vi "boom_monitoring.vi"() -> ()   [LabVIEW 2020]
uses:
  <vilib>/DAQmx/read.llb/DAQmx Read (Analog 1D DBL NChan 1Samp).vi
  <vilib>/DAQmx/create/channels.llb/DAQmx Create Channel (AI-Voltage-Basic).vi
  sub_vi/Timing.llb/getRelativeTime(Host).vi
  <vilib>/DAQmx/miscellaneous.llb/DAQmx Fill In Error Info.vi
  sub_vi/Timing.llb/Timing.lvlib
panel:
  out "error out":errorcluster
  out "logging_state":bool
  in  "logging_cmd":bool
  in  "state":bool
  out "angle_Array":dbl[](array[numeric])
  out "getRelativeTime(sec)":dbl
  out "Waveform Chart":T1(graph)
  in  "zero_set":bool
  in  "Cluster":T2
  out "force":dbl format="%.2f"
  out "displacement":dbl format="%.1f"
  in  "stop":bool
  out "Boolean 6":bool
  out "Boolean 5":bool
  out "Boolean 4":bool
  out "Boolean 3":bool
  out "Boolean 2":bool
  out "Boolean":bool
  out "Angle_7":dbl format="%.1f"
  out "Angle_6":dbl format="%.1f"
  out "Angle_5":dbl format="%.1f"
  out "Angle_4":dbl format="%.1f"
  out "Angle_3":dbl format="%.1f"
  out "Angle_2":dbl format="%.1f"
  out "Angle_1":dbl format="%.1f"
  # "Boom Angle"
  # "Boom1"
  # "Boom2"
  # "Boom3"
  # "Boom4"
  # "Boom5"
  # "Boom6"
  # "Boom7"
  # "kN"
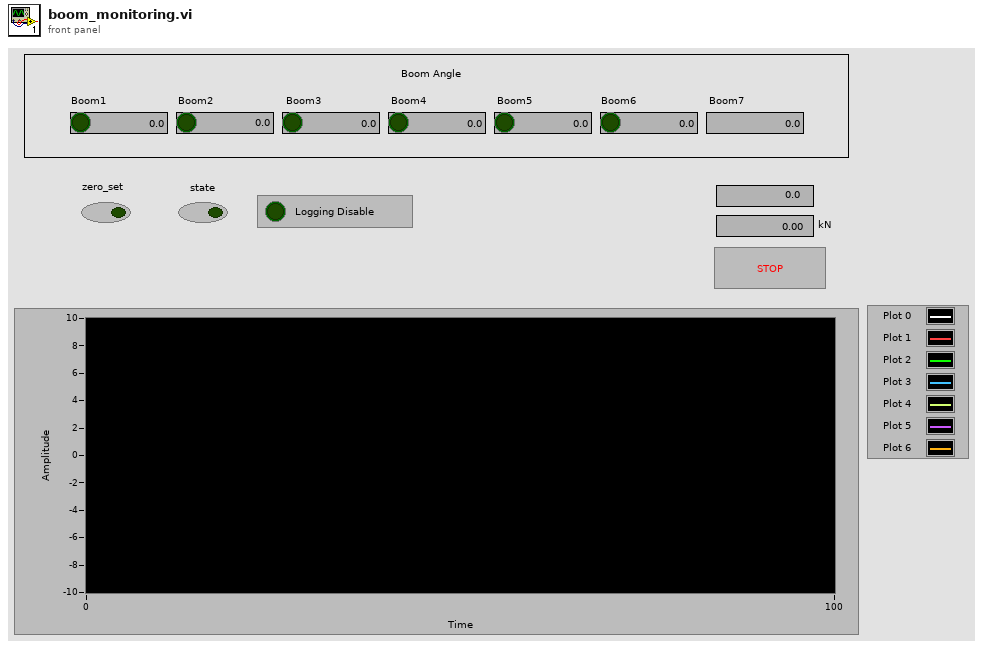
[diagram p1: front panel]
types:
  T1 = cluster{"output_angle(deg)":dbl, "output_angle(deg)":dbl, "output_angle(deg)":dbl, "output_angle(deg)":dbl, "output_angle(deg)":dbl, "output_angle(deg)":dbl, "output_angle(deg)":dbl}
  T2 = cluster{"time(sec)":dbl, "Angle_1(deg)":dbl, "Angle_2(deg)":dbl, "Angle_3(deg)":dbl, "Angle_4(deg)":dbl, "Angle_5(deg)":dbl, "Angle_6(deg)":dbl, "Angle_7(deg)":dbl, "distance(mm)":dbl, "force(kN)":dbl, "state":dbl}
  T3 = enum16{"open", "replace", "create", "open or create", "replace or create", "replace or create with confirmation"}
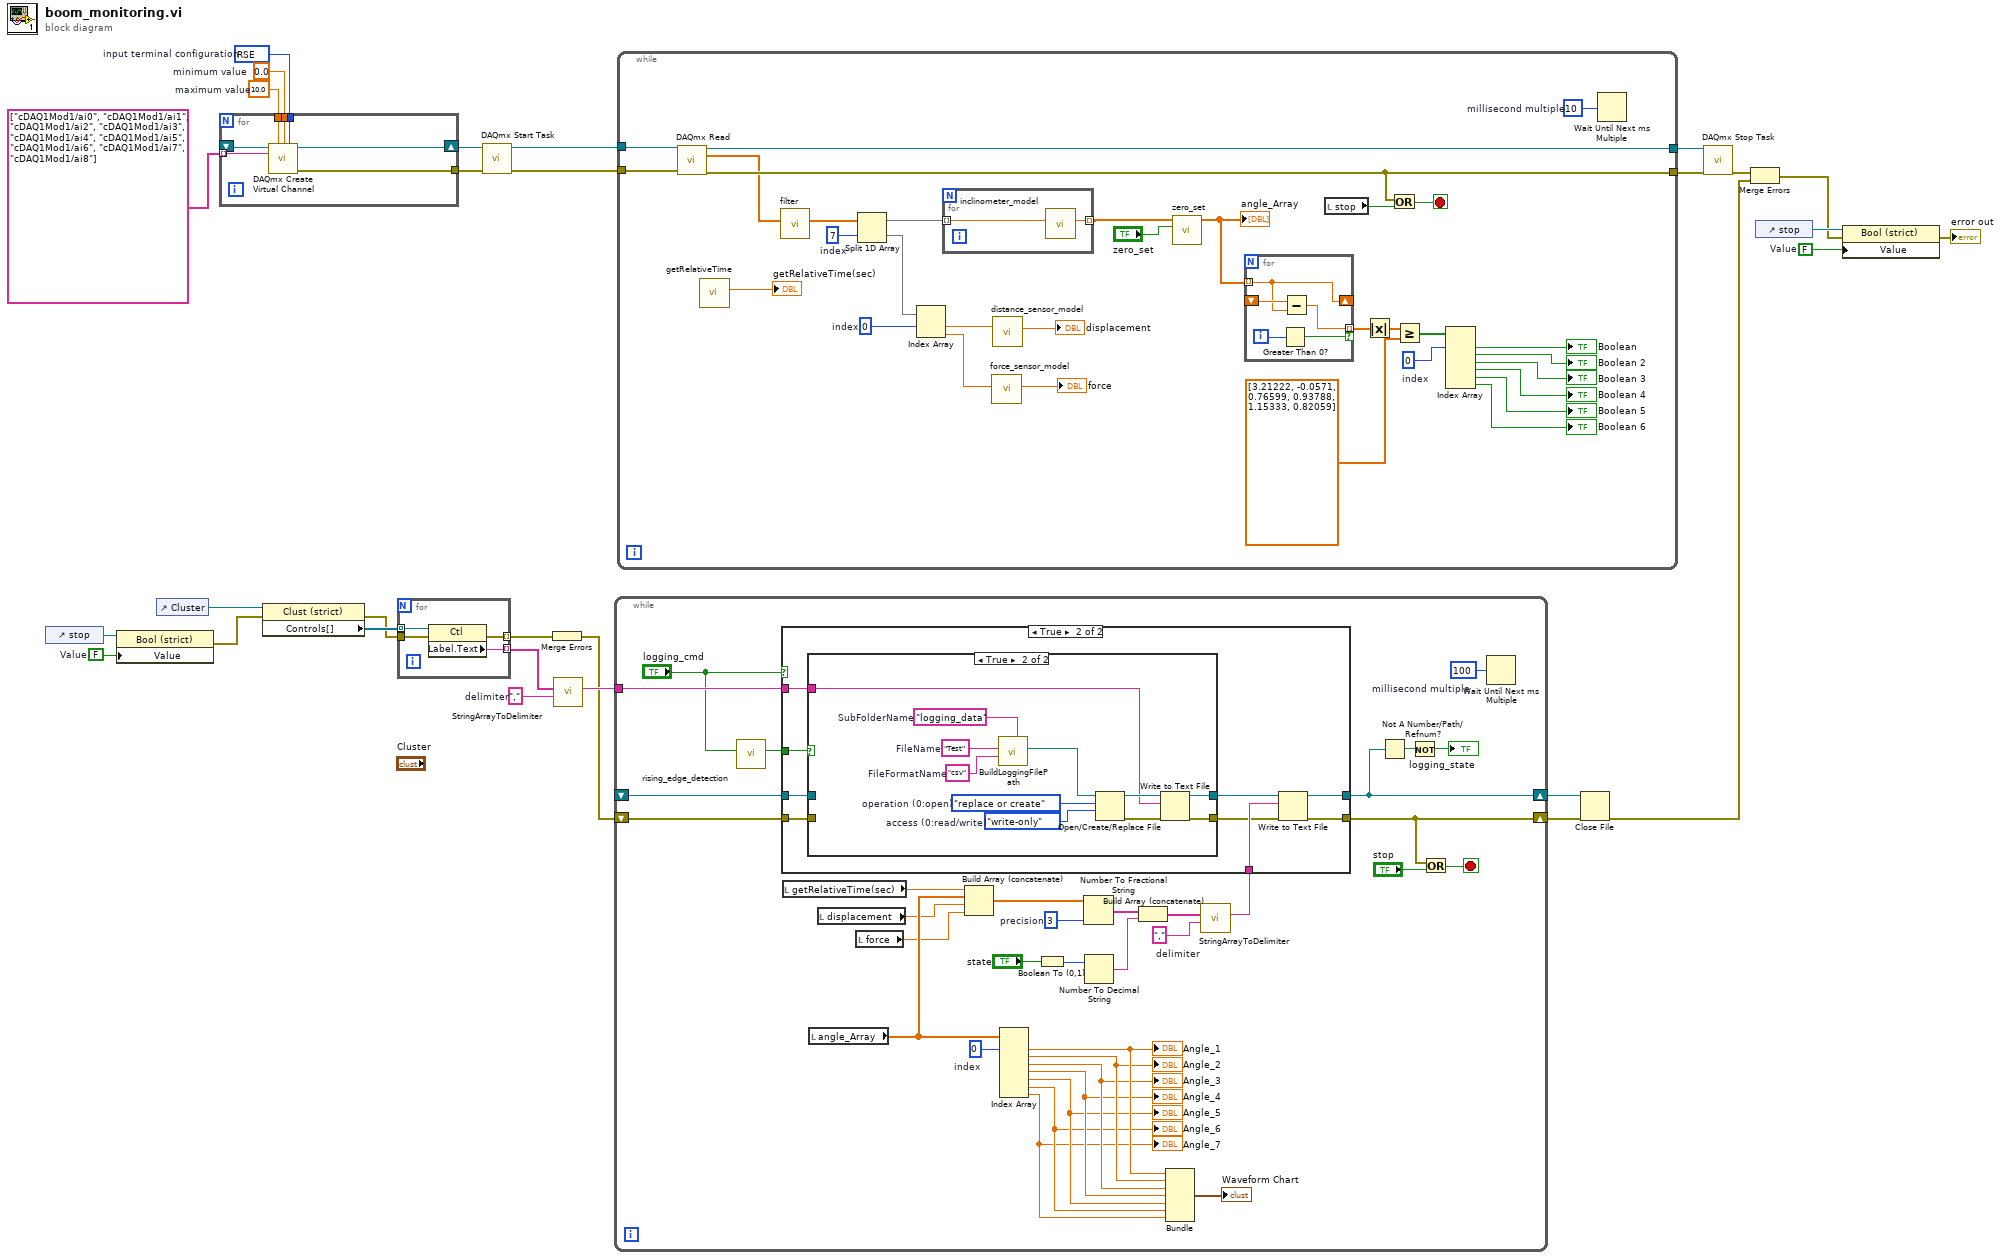
[diagram p0: block diagram]
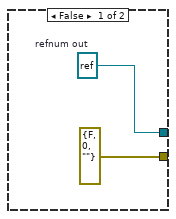
[diagram p2: hidden frame]
diagram:
  w8 = FALSE  # Value
  w11 = FALSE  # Value
  w15 = ","  # delimiter
  w22 = 10.0  # maximum value
  w23 = 0.0  # minimum value
  w24 = 10083 items=["Default"=-1, "RSE"=10083, "NRSE"=10078, "Differential"=10106, "Pseudodifferential"=12529]  # input terminal configuration
  n1 = control-ref of="stop"() -> (w12:refnum<vi>)
  n2 = property class="Bool (strict)"(reference=w12, "Value"=w11) -> (error out=w10:errorcluster)  [unwired: 1 in, 1 out]
  n3 = control-ref of="Cluster"() -> (w19:refnum<vi>)
  n4 = for {
    tunnel: [w35] -> w28
    shift-right: [w36] -> w29
    shift-left: _ -> [w34]
    tunnel: tag[] ["cDAQ1Mod1/ai0", "cDAQ1Mod1/ai1", "cDAQ1Mod1/ai2", "cDAQ1Mod1/ai3", "cDAQ1Mod1/ai4", "cDAQ1Mod1/ai5", "cDAQ1Mod1/ai6", "cDAQ1Mod1/ai7", "cDAQ1Mod1/ai8"] -> [w33] mode=indexing
    tunnel: w24 -> [w32]
    tunnel: w23 -> [w31]
    tunnel: w22 -> [w30]
    n5 = call-poly <vilib>:"DAQmx Create Virtual Channel.vi"("task in"=w34, "maximum value"=w30, "minimum value"=w31, "input terminal configuration"=w32, "physical channels"=w33) -> ("task out"=w36:refnum<k21>, "error out"=w35:errorcluster)  [unwired: 9 in]
  }
  n6 = property class="Clust (strict)"(reference=w19, error in=w10) -> (error out=w17:errorcluster, "Controls[]"=w18:refnum<vi>[])  [unwired: 1 out]
  n7 = for {
    tunnel: w18 -> [w40] mode=indexing
    tunnel: w17 -> [w39]
    tunnel: [w38] -> w16 mode=indexing
    tunnel: [w37] -> w6 mode=indexing
    n8 = property class="Ctl"(reference=w40, error in=w39) -> (error out=w37:errorcluster, "Label.Text"=w38:string)  [unwired: 1 out]
  }
  n9 = call <vilib>:"DAQmx Start Task.vi"("task/channels in"=w29, "error in"=w28) -> ("task out"=w27:refnum<k21>, "error out"=w26:errorcluster)  [unwired: 12 in]
  n10 = Merge Errors(w6) -> (w5:errorcluster)
  n11 = call "StringArrayToDelimiter.vi"("delimiter"=w15, "StringArray"=w16) -> ("String"=w7:string)  [unwired: 9 in]
  n12 = while {
    tunnel: w7 -> [w48]
    shift-right: [w44] -> w14
    shift-left: _ -> [w47]
    shift-right: [w72] -> w13
    shift-left: w5 -> [w46]
    stop <- w71 stop-if-true
    w68 = u32 100  # millisecond multiple
    w70 = 0  # index
    w74 = i16 3  # precision
    w73 = ","  # delimiter
    n13 = call "rising_edge_detection.vi"("input_signal"="logging_cmd") -> ("rising_signal"=w49:bool)  [unwired: 10 in]
    n14 = local read "getRelativeTime(sec)"() -> (w69:dbl)
    n15 = local read "angle_Array"() -> (w59:dbl[])
    n16 = local read "displacement"() -> (w58:dbl)
    n17 = local read "force"() -> (w57:dbl)
    n18 = Build Array (concatenate)(w69, w59, w58, w57) -> (w56:dbl[])
    n19 = Index Array "Index Array"(array=w59, index #1=w70) -> (element #1=w67:dbl, element #2=w66:dbl, element #3=w65:dbl, element #4=w64:dbl, element #5=w63:dbl, element #6=w62:dbl, element #7=w61:dbl)  [unwired: 6 in]
    "Angle_1" <- w67
    "Angle_2" <- w66
    "Angle_3" <- w65
    "Angle_4" <- w64
    "Angle_5" <- w63
    "Angle_6" <- w62
    "Angle_7" <- w61
    n20 = Boolean To (0,1)(Boolean="state") -> (0, 1=w52:i16)
    n21 = Number To Fractional String(number=w56, precision (6)=w74) -> (F-format string=w53:string[])  [unwired: 2 in]
    n22 = Number To Decimal String(number=w52) -> (decimal integer string=w51:string)  [unwired: 1 in]
    n23 = Build Array (concatenate)(w53, w51) -> (w50:string[])
    n24 = Bundle("output_angle(deg)"=w67, "output_angle(deg)"=w66, "output_angle(deg)"=w65, "output_angle(deg)"=w64, "output_angle(deg)"=w63, "output_angle(deg)"=w62, "output_angle(deg)"=w61) -> (→"Waveform Chart":T1)  [unwired: 1 in]
    n25 = call "StringArrayToDelimiter.vi"("delimiter"=w73, "StringArray"=w50) -> ("String"=w55:string)  [unwired: 9 in]
    n26 = case shown="True" "logging_cmd" {
      tunnel: [w76 w85] -> w44
      tunnel: [errorcluster {"status"=FALSE, "code"=0, "source"=""} ("error out") w84] -> w72
      tunnel: w55 -> [_ w83]
      tunnel: w49 -> [_ w82]
      tunnel: w48 -> [_ w81]
      tunnel: w47 -> [_ w78]
      tunnel: w46 -> [_ w77]
      frame False {
        w76 = refnum<file> refnum  # refnum out
      }
      frame True {
        n27 = case shown="True" w82 {
          tunnel: w81 -> [_ w90]
          tunnel: [w87 w89] -> w80
          tunnel: [w86 w88] -> w79
          tunnel: w78 -> [w87 _]
          tunnel: w77 -> [w86 _]
          frame False {
          }
          frame True {
            w94 = "csv"  # FileFormatName
            w95 = "logging_data"  # SubFolderName
            w93 = "Test"  # FileName
            w92 = enum16{"read/write", "read-only", "write-only"}."write-only"  # access (0:read/write)
            w91 = T3."replace or create"  # operation (0:open)
            n28 = call "BuildLoggingFilePath.vi"("SubFolderName"=w95, "FileFormatName"=w94, "FileName"=w93) -> ("appended path"=w97:path)  [unwired: 8 in]
            n29 = Open/Create/Replace File(file path (use dialog)=w97, operation (0:open)=w91, access (0:read/write)=w92) -> (refnum out=w96:refnum<file>, error out=w98:errorcluster)  [unwired: 3 in, 1 out]
            n30 = Write to Text File(file (use dialog)=w96, text=w90, error in=w98) -> (refnum out=w89:refnum<file>, error out=w88:errorcluster)  [unwired: 1 in, 1 out]
          }
        }
        n31 = Write to Text File(file (use dialog)=w80, text=w83, error in=w79) -> (refnum out=w85:refnum<file>, error out=w84:errorcluster)  [unwired: 1 in, 1 out]
      }
    }
    n32 = Not A Number/Path/Refnum?(number/path/refnum=w44) -> (NaN/Path/Refnum?=w43:bool)
    n33 = Not(x=w43) -> (.not. x?=→"logging_state":bool)
    n34 = Or(x=w72, y="stop") -> (x .or. y?=w71:bool)
    n35 = Wait Until Next ms Multiple(millisecond multiple=w68) -> ()  [unwired: 1 out]
  }
  n36 = while {
    tunnel: w27 -> [w130]
    tunnel: w26 -> [w129]
    tunnel: [w128] -> w21
    tunnel: [w122] -> w20
    stop <- w121 stop-if-true
    w104 = 0  # index
    w124 = 0  # index
    w126 = 7  # index
    w127 = u32 10  # millisecond multiple
    n37 = call-poly <vilib>:"DAQmx Read.vi"("task/channels in"=w130, "error in"=w129) -> ("task out"=w128:refnum<k21>, "data"=w114:dbl[], "error out"=w122:errorcluster)  [unwired: 11 in]
    n38 = call-poly "getRelativeTime.vi"() -> ("getRelativeTime(sec)"=→"getRelativeTime(sec)":dbl)  [unwired: 11 in]
    n39 = call "filter.vi"("data_input"=w114) -> ("appended array"=w115:dbl[])  [unwired: 10 in]
    n40 = Split 1D Array(array=w115, index=w126) -> (first subarray=w102:dbl[], second subarray=w125:dbl[])
    n41 = Index Array "Index Array"(array=w125, index #1=w124) -> (element #1=w120:dbl, element #2=w119:dbl)  [unwired: 1 in]
    n42 = for {
      tunnel: [w137] -> w101 mode=indexing
      tunnel: w102 -> [w136] mode=indexing
      n43 = call "inclinometer_model.vi"("input_signal(V)"=w136) -> ("output_angle(deg)"=w137:dbl)  [unwired: 10 in]
    }
    n44 = call "force_sensor_model.vi"("voltage_input"=w119) -> ("force_output"=→"force":dbl)  [unwired: 10 in]
    n45 = call "distance_sensor_model.vi"("voltage_input"=w120) -> ("distance_output"=→"displacement":dbl)  [unwired: 10 in]
    n46 = call "zero_set.vi"("zero_set"="zero_set", "data_input"=w101) -> ("data_output"=w100:dbl[])  [unwired: 9 in]
    "angle_Array" <- w100
    n47 = for {
      tunnel: w100 -> [w134] mode=indexing
      shift-right: [w134] -> _
      shift-left: _ -> [w135]
      tunnel: [w133] -> w113 mode=indexing if=w131
      i -> [w132]
      n48 = Greater Than 0?(x=w132) -> (x > 0?=w131:bool)
      n49 = Subtract(x=w135, y=w134) -> (x-y=w133:dbl)
    }
    n50 = local read "stop"() -> (w99:bool)
    n51 = Absolute Value(x=w113) -> (abs(x)=w105:dbl[])
    n52 = Or(x=w122, y=w99) -> (x .or. y?=w121:bool)
    n53 = Greater Or Equal?(x=w105, y=dbl[] [3.21222, -0.0571, 0.76599, 0.93788, 1.15333, 0.82059]) -> (x >= y?=w112:bool[])
    n54 = Index Array "Index Array"(array=w112, index #1=w104) -> (element #1=→"Boolean":bool, element #2=→"Boolean 2":bool, element #3=→"Boolean 3":bool, element #4=→"Boolean 4":bool, element #5=→"Boolean 5":bool, element #6=→"Boolean 6":bool)  [unwired: 5 in]
    n55 = Wait Until Next ms Multiple(millisecond multiple=w127) -> ()  [unwired: 1 out]
  }
  n56 = Close File(refnum=w14, error in=w13) -> (error out=w4:errorcluster)  [unwired: 1 out]
  n57 = call <vilib>:"DAQmx Stop Task.vi"("task/channels in"=w21, "error in"=w20) -> ("error out"=w3:errorcluster)  [unwired: 12 in, 1 out]
  n58 = Merge Errors(w3, w4) -> (w2:errorcluster)
  n59 = control-ref of="stop"() -> (w9:refnum<vi>)
  n60 = property class="Bool (strict)"(reference=w9, error in=w2, "Value"=w8) -> (error out=→"error out":errorcluster)  [unwired: 1 out]
